vi "TestEngineerOverview.vi"() -> ()   [LabVIEW 2020]
uses:
  <vilib>/Utility/file.llb/Read Delimited Spreadsheet (DBL).vi
  Controls/MotorSelection.ctl
  Controls/Automated Tests.ctl
panel:
  in  "Tab Control":enum32{"Test Execution", "Page 2"}(tab)
  in  "PauseTest":bool
  in  "StopTest":bool
  in  "StartTest":bool
  in  "Select automated test":T1
  in  "Select Motor":T2
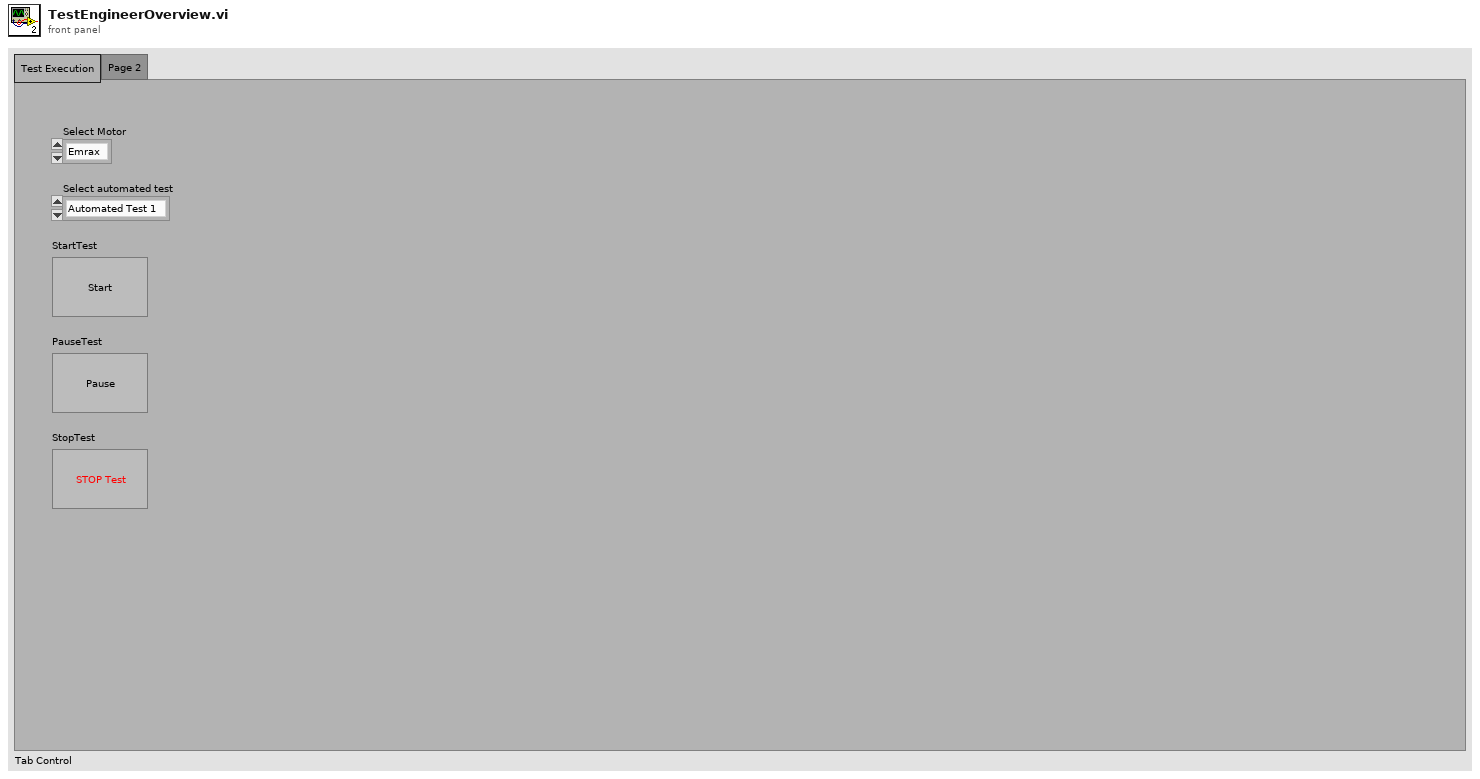
[diagram p1: front panel]
types:
  T1 = typedef "Automated Tests.ctl" = enum16{"Automated Test 1", "Automated Test 2", "Automated Test 3"}
  T2 = typedef "MotorSelection.ctl" = enum16{"Emrax", "Hacker", "Saluqi"}
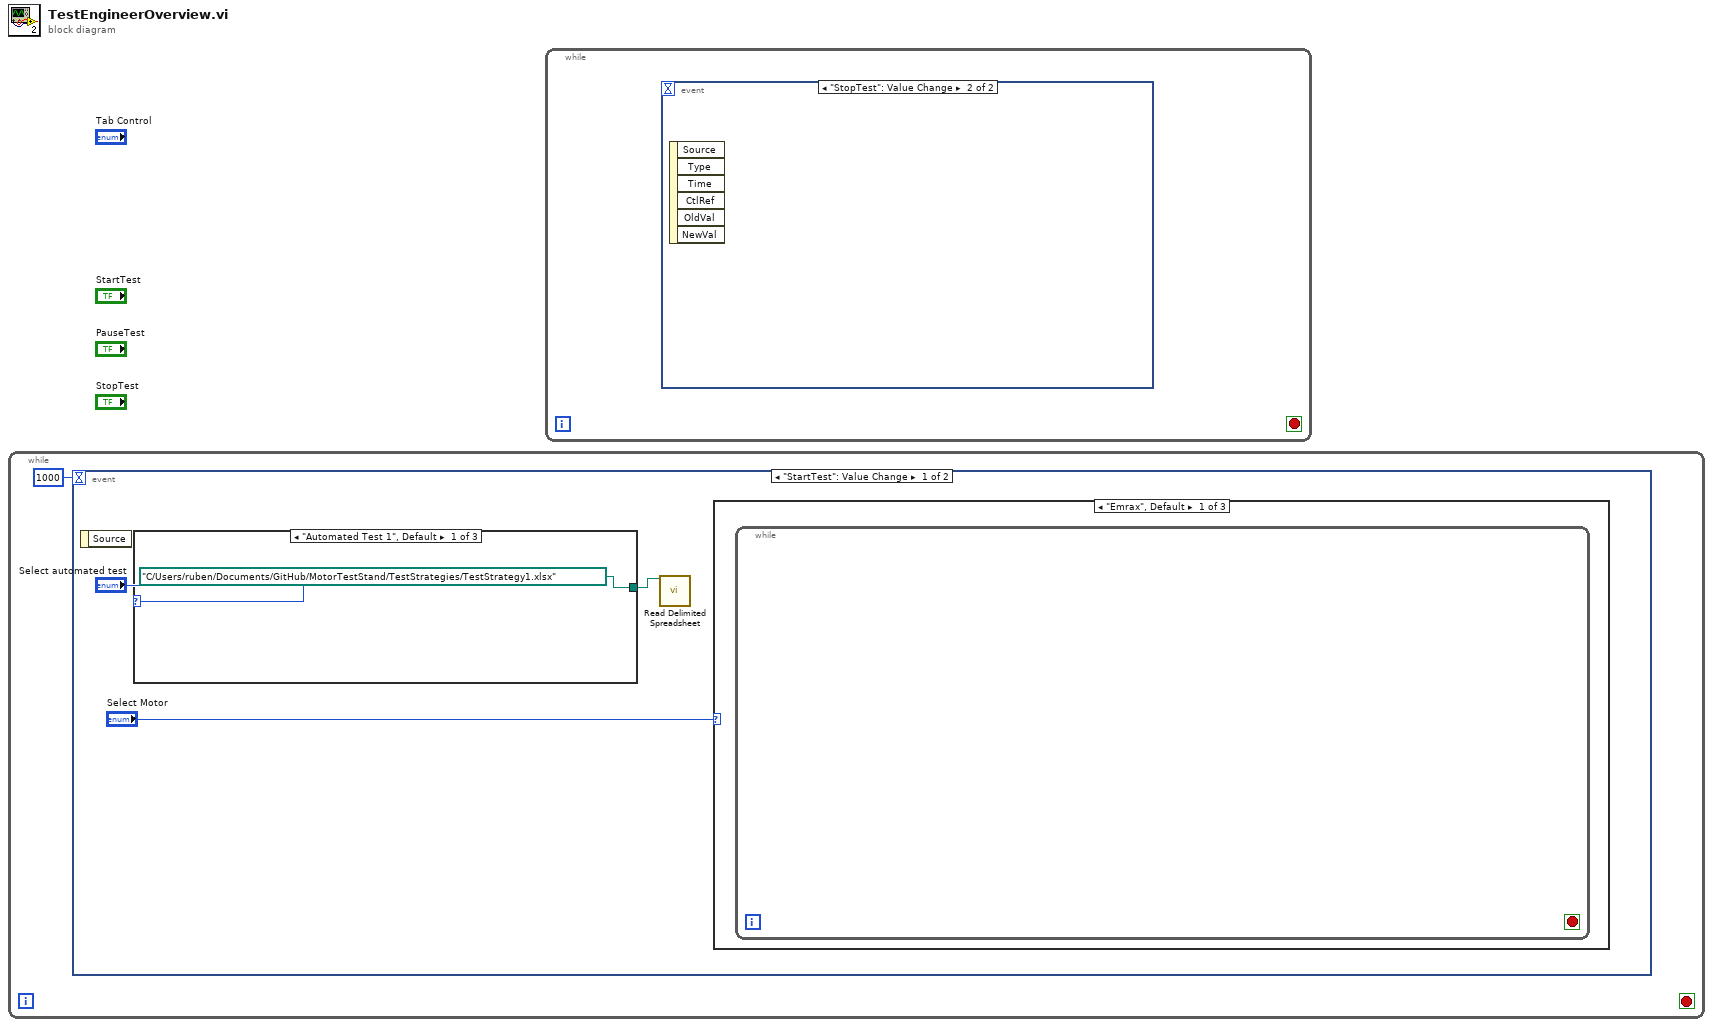
[diagram p0: block diagram]
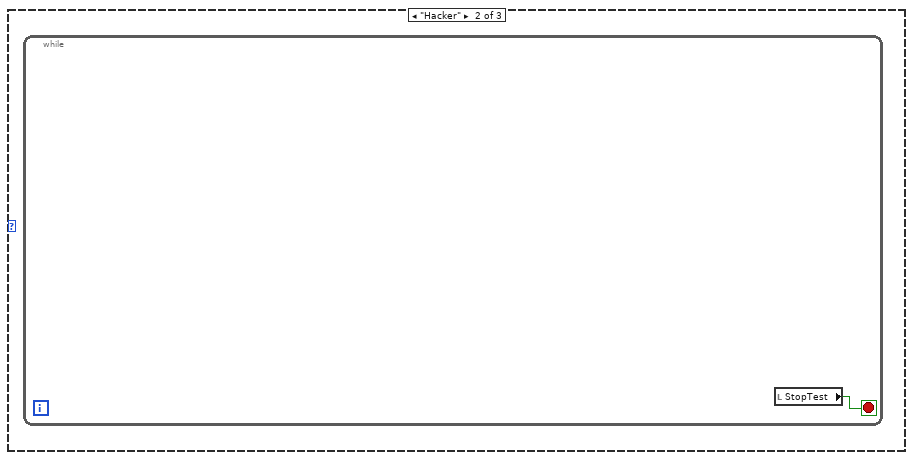
[diagram p4: hidden frame]
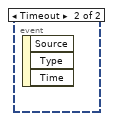
[diagram p6: hidden frame]
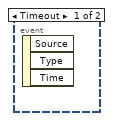
[diagram p7: hidden frame]
diagram:
  n1 = while {
    stop <- _ stop-if-true
    n2 = event shown="[0] \"StartTest\": Value Change" {
      selector: _ -> [_ _]
      dyn-events: _ -> [_ _]
      timeout: 1000 -> [_ _]
      event "StartTest": Value Change {
        n3 = event-data() -> ()  [unwired: 1 in, 1 out]
        n4 = case shown="\"Automated Test 1\", Default" "Select automated test" {
          tunnel: [path "C:/Users/ruben/Documents/GitHub/MotorTestStand/TestStrategies/TestStrategy1.xlsx" ("Path") _ _] -> w2
          frame "Automated Test 1", Default {
          }
          frame "Automated Test 2" {
          }
          frame "Automated Test 3" {
          }
        }
        n5 = call-poly <vilib>:"Read Delimited Spreadsheet.vi"("file path (dialog if empty)"=w2) -> ()  [unwired: 9 in, 6 out]
        n6 = case shown="\"Emrax\", Default" "Select Motor" {
          frame "Emrax", Default {
            n7 = while {
              stop <- _ stop-if-true
            }
          }
          frame "Hacker" {
            n8 = while {
              stop <- w6 stop-if-true
              n9 = local read "StopTest"() -> (w6:bool)
            }
          }
          frame "Saluqi" {
          }
        }
      }
      event Timeout {
        n10 = event-data() -> ()  [unwired: 1 in, 3 out]
      }
    }
  }
  n11 = while {
    stop <- _ stop-if-true
    n12 = event shown="[1] \"StopTest\": Value Change" {
      selector: _ -> [_ _]
      dyn-events: _ -> [_ _]
      timeout: _ -> [_ _]
      event Timeout {
        n13 = event-data() -> ()  [unwired: 1 in, 3 out]
      }
      event "StopTest": Value Change {
        n14 = event-data() -> ()  [unwired: 1 in, 6 out]
      }
    }
  }
